vi "Analog Login.vi"() -> (1 "Boolean 2":bool caption="Boolean", 2 "Password 2":string, 3 "User Name 2":string)   [LabVIEW 2017]
panel:
  in  "Login":bool caption="Boolean"
  in  "Password":string
  in  "User Name":string
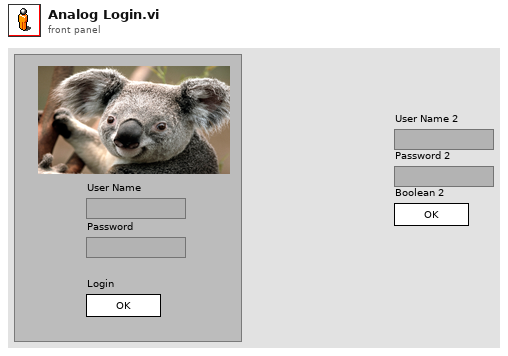
[diagram p1: front panel]
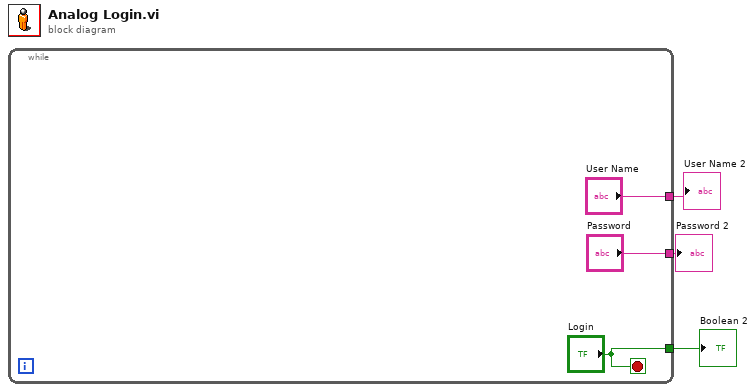
[diagram p0: block diagram]
diagram:
  n1 = while {
    tunnel: ["User Name"] -> w3
    tunnel: ["Password"] -> w2
    tunnel: ["Login"] -> w1
    stop <- "Login" stop-if-true
  }
  "User Name 2" <- w3
  "Password 2" <- w2
  "Boolean 2" <- w1
